vi "Disabled.vi"(7 "Robot Mode":T3, 10 "Match Info":T2={"Autonomous Elapsed Seconds"=0.0, "TeleOp Elapsed Seconds"=0.0, "Disabled Elapsed Seconds"=0.0, "Visited Autonomous"=FALSE, "Visited TeleOp"=FALSE, "Visited Disabled"=FALSE, "Autonomous Settings"={"Autonomous Style"=enum."Independent", "VI Refnum"=refnum}}, 11 "Call Context":T4) -> ()   [LabVIEW 2011]
doc: "This VI is called each time a disabled packet is received from the DS. It is often used to prepare for the next robot mode, to calibrate sensors, etc."
uses:
  <vilib>/Rock Robotics/WPI/DriverStation/WPI_DriverStationDerivedRobotMode.ctl
  <vilib>/Rock Robotics/WPI/DriverStation/WPI_DriverStationRobotMode.ctl
  <vilib>/Rock Robotics/WPI/DriverStation/WPI_DriverStationMatch Info.ctl
  <vilib>/Rock Robotics/WPI/Joystick/WPI_JoystickButtonState.ctl
  Robot Global Data.vi
panel:
  in  "Allow Change":bool
  out "Buttons 2":T1
  out "Buttons":T1
  in  "Refresh":bool
  in  "Auton File":dbl
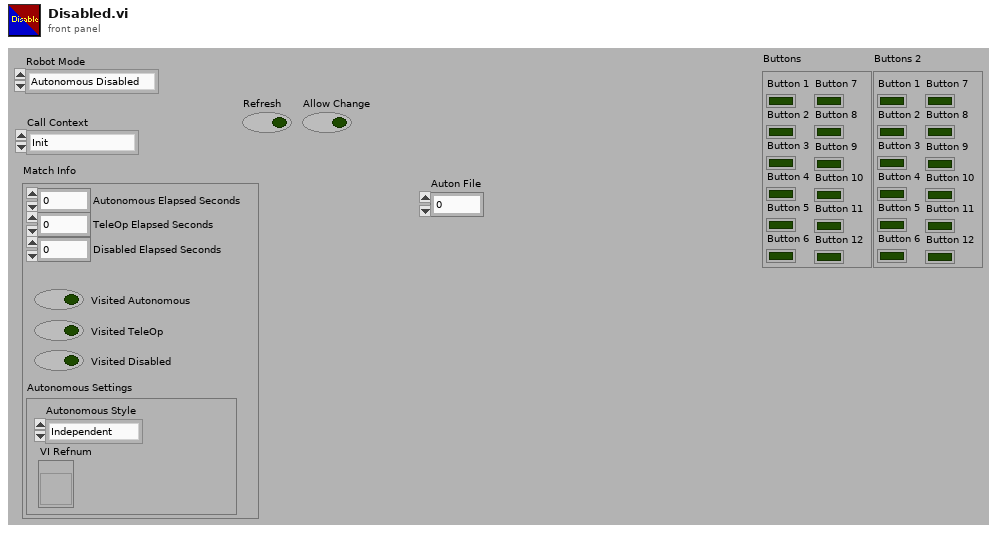
[diagram p1: front panel]
types:
  T1 = typedef "WPI_JoystickButtonState.ctl" = cluster{"Button 1":bool, "Button 2":bool, "Button 3":bool, "Button 4":bool, "Button 5":bool, "Button 6":bool, "Button 7":bool, "Button 8":bool, "Button 9":bool, "Button 10":bool, "Button 11":bool, "Button 12":bool}
  T2 = typedef "WPI_DriverStationMatch Info.ctl" = cluster{"Autonomous Elapsed Seconds":dbl, "TeleOp Elapsed Seconds":dbl, "Disabled Elapsed Seconds":dbl, "Visited Autonomous":bool, "Visited TeleOp":bool, "Visited Disabled":bool, "Autonomous Settings":cluster{"Autonomous Style":enum16{"Iterative", "Independent"}, "VI Refnum":refnum<vi>}}
  T3 = typedef "WPI_DriverStationRobotMode.ctl" = enum16{"Autonomous Disabled", "Autonomous Enabled", "Teleop Disabled", "Teleop Enabled", "Timeout", "Finish"}
  T4 = typedef "WPI_DriverStationDerivedRobotMode.ctl" = enum16{"Init", "Execute", "Stop"}
  T5 = typedef "WPI_JoystickDevRef.ctl" = cluster{"Device":T6}
  T6 = typedef "WPI_JoystickDeviceEnum.ctl" = enum16{"USB 1", "USB 2", "USB 3", "USB 4", "Kinect 1", "Kinect 2"}
  T7 = typedef "WPI_EncoderDevRef.ctl" = cluster{"DevStatus":errorcluster, "EncoderIndex":T8, "CounterIndex":T9, "DistancePerCount":dbl, "Decoding Type":T10}
  T8 = typedef "FPGA_EncoderIdx.ctl" = enum8{"Enc 0", "Enc 1", "Enc 2", "Enc 3", "Invalid"}
  T9 = typedef "FPGA_CounterCtrSystemIndex.ctl" = enum8{"Ctr 0", "Ctr 1", "Ctr 2", "Ctr 3", "Ctr 4", "Ctr 5", "Ctr 6", "Ctr 7", "Invalid"}
  T10 = typedef "WPI_EncoderType.ctl" = enum16{"1x", "2x", "4x"}
  T11 = typedef "WPI_GyroDevRef.ctl" = cluster{"DevStatus":errorcluster, "Analog Module":T12, "Analog Channel":T13, "Offset":dbl, "Gain (VoltsPerDegree/Second)":dbl}
  T12 = typedef "FPGA_TypedefAnalogModule.ctl" = enum16{"Analog Module 1", "Analog Module 2"}
  T13 = typedef "FPGA_AIChannel.ctl" = enum8{"AI 1", "AI 2", "AI 3", "AI 4", "AI 5", "AI 6", "AI 7", "AI 8", "Invalid"}
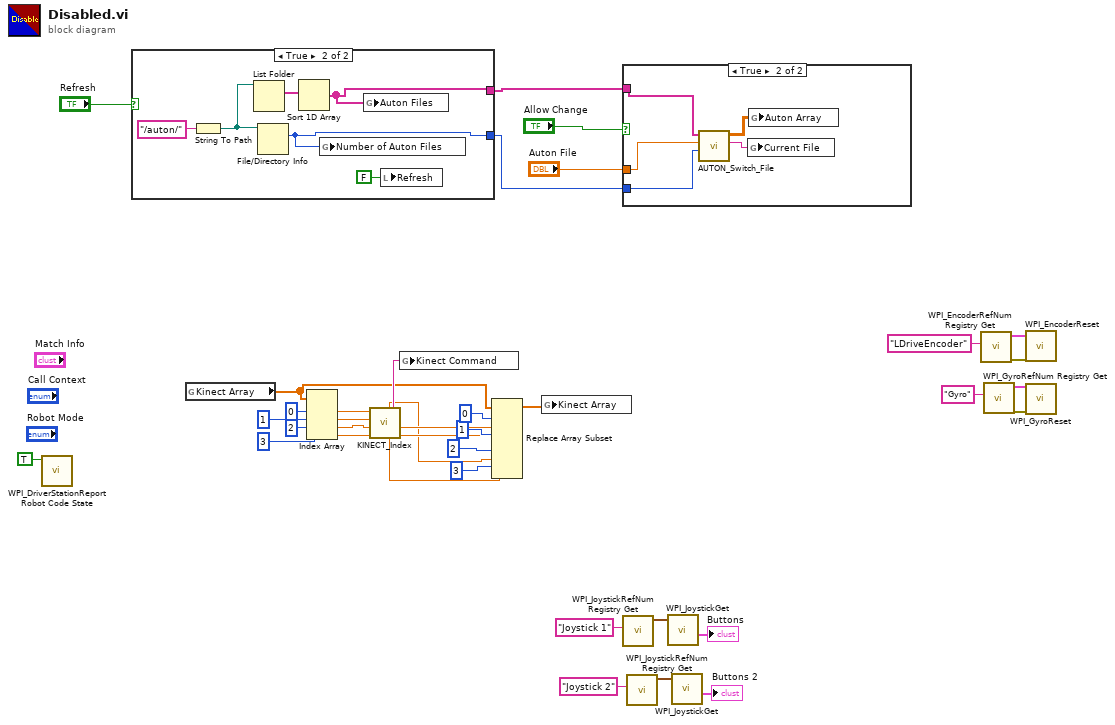
[diagram p0: block diagram]
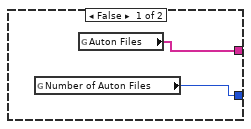
[diagram p3: hidden frame]
diagram:
  n1 = call <vilib>:"WPI_DriverStationReport Robot Code State.vi"("Disabled"=TRUE ("Autonomous")) -> ()  [unwired: 10 in, 1 out]
  n2 = case shown="True" "Refresh" {
    tunnel: [w38 w42] -> w7
    tunnel: [w39 w41] -> w8
    frame False {
      n3 = global read "Robot Global Data.vi" "Number of Auton Files"() -> (w38:i64)
      n4 = global read "Robot Global Data.vi" "Auton Files"() -> (w39:string[])
    }
    frame True {
      n5 = String To Path(string="/auton/") -> (path=w44:path)
      n6 = List Folder(path=w44) -> (filenames=w43:string[])  [unwired: 1 in, 5 out]
      n7 = File/Directory Info(path=w44) -> (size=w42:i64)  [unwired: 1 in, 6 out]
      n8 = Sort 1D Array(array=w43) -> (sorted array=w41:string[])
      n9 = global write "Robot Global Data.vi" "Number of Auton Files"(w42) -> ()
      n10 = global write "Robot Global Data.vi" "Auton Files"(w41) -> ()
      n11 = local write "Refresh"(FALSE ("Refresh")) -> ()
    }
  }
  n12 = global read "Robot Global Data.vi" "Kinect Array"() -> (w27:dbl[])
  n13 = Index Array(array=w27, index #1=0 ("index"), index #2=1 ("index"), index #3=2 ("index"), index #4=3 ("index")) -> (element #1=w31:dbl, element #2=w30:dbl, element #3=w29:dbl, element #4=w28:dbl)
  n14 = call "KINECT_Index.vi"("Arm Drive Min in (Reverse)"=w28, "Arm Drive Max in (Forward)"=w29, "Z Wrist Left"=w30, "Z Wrist Right"=w31) -> ("Z Wrist Left"=w23:sgl, "Z Wrist Right"=w25:sgl, "Kinect Command"=w36:string, "Arm Drive Min out (Reverse)"=w19:dbl, "Arm Drive Max out (Forward)"=w20:dbl)  [unwired: 3 in]
  n15 = global write "Robot Global Data.vi" "Kinect Command"(w36) -> ()
  n16 = Replace Array Subset(array=w27, new element #1=w25, index #1=0 ("index"), new element #2=w23, index #2=1 ("index"), new element #3=w20, index #3=2 ("index"), new element #4=w19, index #4=3 ("index")) -> (w18:dbl[])
  n17 = global write "Robot Global Data.vi" "Kinect Array"(w18) -> ()
  n18 = case shown="True" "Allow Change" {
    tunnel: "Auton File" -> [_ w48]
    tunnel: w8 -> [_ w47]
    tunnel: w7 -> [_ w46]
    frame False {
    }
    frame True {
      n19 = call "AUTON_Switch_File.vi"("Number of Auton Files"=w46, "Auton File"=w48, "Auton Files"=w47) -> ("Current File"=w49:string, "Auton Array"=w50:dbl[][])  [unwired: 7 in]
      n20 = global write "Robot Global Data.vi" "Current File"(w49) -> ()
      n21 = global write "Robot Global Data.vi" "Auton Array"(w50) -> ()
    }
  }
  n22 = call <vilib>:"WPI_JoystickRefNum Registry Get.vi"("refnum name"="Joystick 1") -> ("JoystickDevRef"=w16:T5)  [unwired: 9 in, 1 out]
  n23 = call <vilib>:"WPI_JoystickRefNum Registry Get.vi"("refnum name"="Joystick 2") -> ("JoystickDevRef"=w13:T5)  [unwired: 9 in, 1 out]
  n24 = call <vilib>:"WPI_JoystickGet.vi"("JoystickDevRef"=w16) -> ("Buttons"=→"Buttons":T1)  [unwired: 4 in, 2 out]
  n25 = call <vilib>:"WPI_JoystickGet.vi"("JoystickDevRef"=w13) -> ("Buttons"=→"Buttons 2":T1)  [unwired: 4 in, 2 out]
  n26 = call <vilib>:"WPI_EncoderRefNum Registry Get.vi"("refnum name"="LDriveEncoder") -> ("error out"=w6:errorcluster, "EncoderDevRef"=w5:T7)  [unwired: 9 in]
  n27 = call <vilib>:"WPI_GyroRefNum Registry Get.vi"("refnum name"="Gyro") -> ("error out"=w3:errorcluster, "GyroDevRef"=w4:T11)  [unwired: 9 in]
  n28 = call <vilib>:"WPI_EncoderReset.vi"("error in (no error)"=w6, "EncoderDevRef"=w5) -> ()  [unwired: 8 in, 2 out]
  n29 = call <vilib>:"WPI_GyroReset.vi"("error in (no error)"=w3, "GyroDevRef"=w4) -> ()  [unwired: 8 in, 2 out]
